vi "parse_header_a.vi"(11 "data in":string) -> (0 "payload len code":u8, 1 "fin?":u8, 2 "opcode":T1 items=["continue"=0, "text"=1, "binary"=2, "hangup"=8, "ping"=9, "pong"=10], 3 "mask?":u8)   [LabVIEW 2019, in "WebSocket Server Toolkit.lvlib"]
uses:
  WebSocket Server Toolkit.lvlib
  types/opcode.ctl
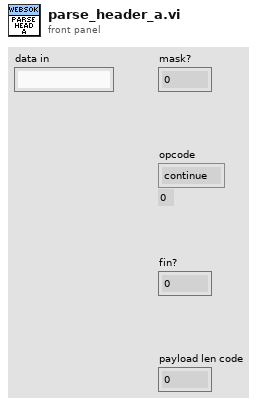
[diagram p1: front panel]
types:
  T1 = typedef "WebSocket Server Toolkit.lvlib/opcode.ctl" = u8
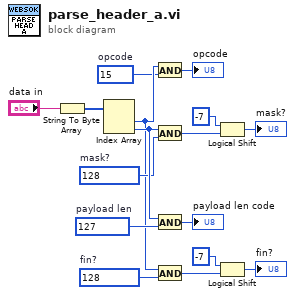
[diagram p0: block diagram]
diagram:
  w16 = u8 127  # payload len
  w14 = u8 128  # mask?
  w12 = u8 15  # opcode
  w10 = u8 128  # fin?
  n1 = String To Byte Array(string="data in") -> (unsigned byte array=w11:u8[])
  n2 = Index Array(array=w11) -> (element #1=w13:u8, element #2=w15:u8)  [unwired: 2 in]
  n3 = And(x=w13, y=w12) -> (x .and. y?=→"opcode":u8)
  n4 = And(x=w15, y=w14) -> (x .and. y?=w2:u8)
  n5 = And(x=w15, y=w16) -> (x .and. y?=→"payload len code":u8)
  n6 = And(x=w13, y=w10) -> (x .and. y?=w8:u8)
  n7 = Logical Shift(y=i16 -7, x=w2) -> (x << y=→"mask?":u8)
  n8 = Logical Shift(y=i16 -7, x=w8) -> (x << y=→"fin?":u8)
